vi "SubVI server withdraw.vi"(9 "before match":string, 10 "after match":string, 11 "appended path":path) -> (3 "String":string)   [LabVIEW 2020]
uses:
  <vilib>/Utility/file.llb/Read Delimited Spreadsheet (string).vi
  <vilib>/Utility/file.llb/Write Delimited Spreadsheet (string).vi
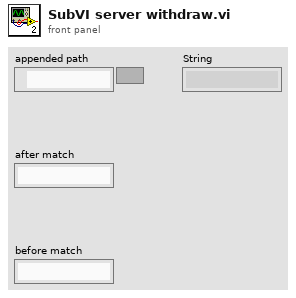
[diagram p1: front panel]
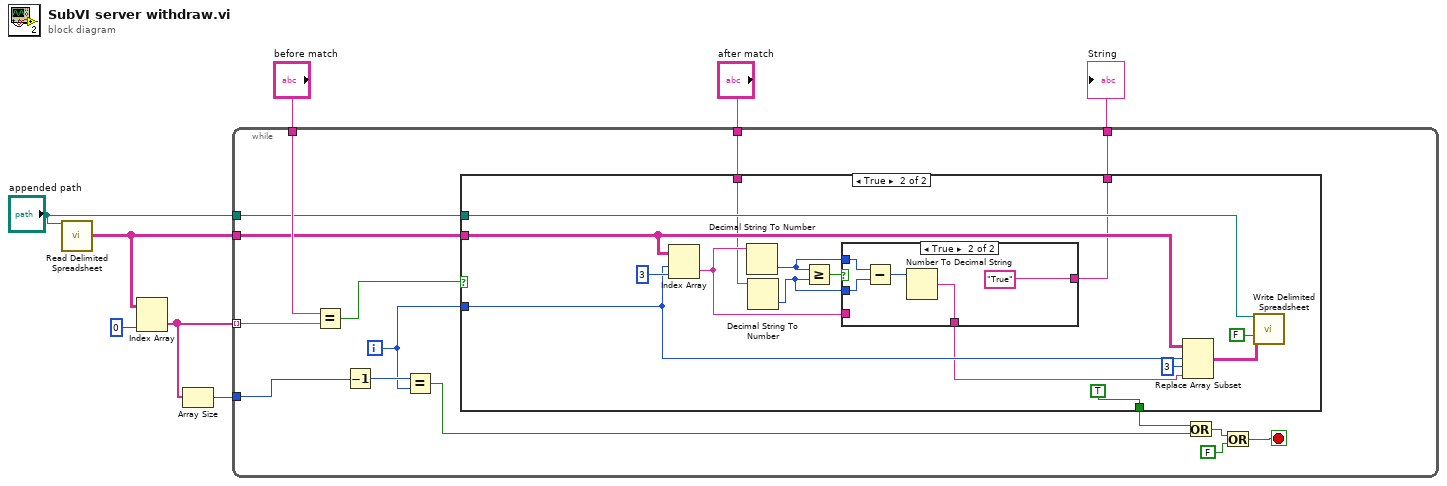
[diagram p0: block diagram]
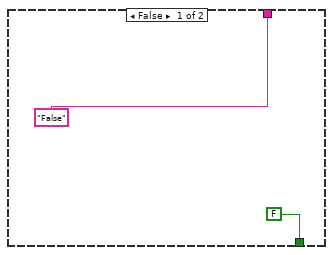
[diagram p2: hidden frame]
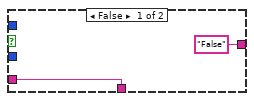
[diagram p3: hidden frame]
diagram:
  n1 = call-poly <vilib>:"Read Delimited Spreadsheet.vi"("file path (dialog if empty)"="appended path") -> ("all rows"=w3:string[][])  [unwired: 9 in, 5 out]
  n2 = Index Array "Index Array"(array=w3, index (col)=0 ("disabled index (col)")) -> (element=w2:string[])  [unwired: 1 in]
  n3 = Array Size(array=w2) -> (size(s)=w1:i32)
  n4 = while {
    tunnel: w3 -> [w18]
    tunnel: w2 -> [w15] mode=indexing
    tunnel: "before match" -> [w20]
    tunnel: w1 -> [w17]
    tunnel: "appended path" -> [w14]
    tunnel: [w13] -> w7
    tunnel: "after match" -> [w12]
    i -> [w16]
    stop <- w21 stop-if-true
    n5 = Equal?(x=w20, y=w15) -> (x = y?=w19:bool)
    n6 = Decrement(x=w17) -> (x-1=w22:i32)
    n7 = Equal?(x=w22, y=w16) -> (x = y?=w10:bool)
    n8 = case shown="True" w19 {
      tunnel: w18 -> [_ w37]
      tunnel: w16 -> [_ w28]
      tunnel: w14 -> [_ w40]
      tunnel: ["False" w35] -> w13
      tunnel: w12 -> [_ w29]
      tunnel: [FALSE TRUE] -> w9
      frame False {
      }
      frame True {
        n9 = Index Array(array=w37, index (row)=w28, index (col)=3 ("disabled index (col)")) -> (element=w30:string)
        n10 = Decimal String To Number(string=w30) -> (number=w33:i32)  [unwired: 2 in, 1 out]
        n11 = Decimal String To Number(string=w29) -> (number=w32:i32)  [unwired: 2 in, 1 out]
        n12 = Greater Or Equal?(x=w33, y=w32) -> (x >= y?=w34:bool)
        n13 = case shown="True" w34 {
          tunnel: ["False" "True"] -> w35
          tunnel: w33 -> [_ w47]
          tunnel: w32 -> [_ w46]
          tunnel: [w41 w44] -> w26
          tunnel: w30 -> [w41 _]
          frame False {
          }
          frame True {
            n14 = Subtract(x=w47, y=w46) -> (x-y=w45:i32)
            n15 = Number To Decimal String(number=w45) -> (decimal integer string=w44:string)  [unwired: 1 in]
          }
        }
        n16 = Replace Array Subset(array=w37, new element=w26, index (row)=w28, index (col)=3 ("disabled index (col)")) -> (w39:string[][])
        n17 = call-poly <vilib>:"Write Delimited Spreadsheet.vi"("file path (dialog if empty)"=w40, "2D data"=w39, "append to file? (new file:F)"=FALSE) -> ()  [unwired: 11 in, 2 out]
      }
    }
    n18 = Or(x=w9, y=w10) -> (x .or. y?=w11:bool)
    n19 = Or(x=w11, y=FALSE) -> (x .or. y?=w21:bool)
  }
  "String" <- w7
